vi "LV-Term UI.vi"(11 "LV-Term App In":refnum<class "LV-Term App.lvclass">) -> (3 "LV-Term App":refnum<class "LV-Term App.lvclass">)   [LabVIEW 2020, in "LV-Term App.lvclass"]
uses:
  LV-Term App.lvclass
  UI State.ctl
  LV-Term App.lvclass/LV-Term App.ctl
  Terminal/Terminal/Terminal.lvclass
  C:/Program Files (x86)/National Instruments/LabVIEW 2020/vi.lib/IlluminatedG/IG OOPanel/OOPanel/Panel/Panel.lvclass
  <vilib>/IlluminatedG/IG OOPanel/OOPanel/Manager/Manager.lvclass
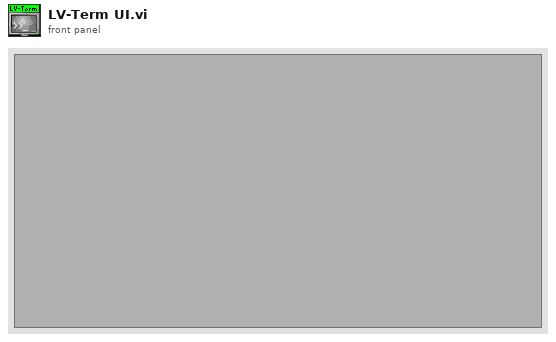
[diagram p1: front panel]
types:
  T1 = typedef "LV-Term App.lvclass/UI State.ctl" = enum16{"Init", "Run", "Close"}
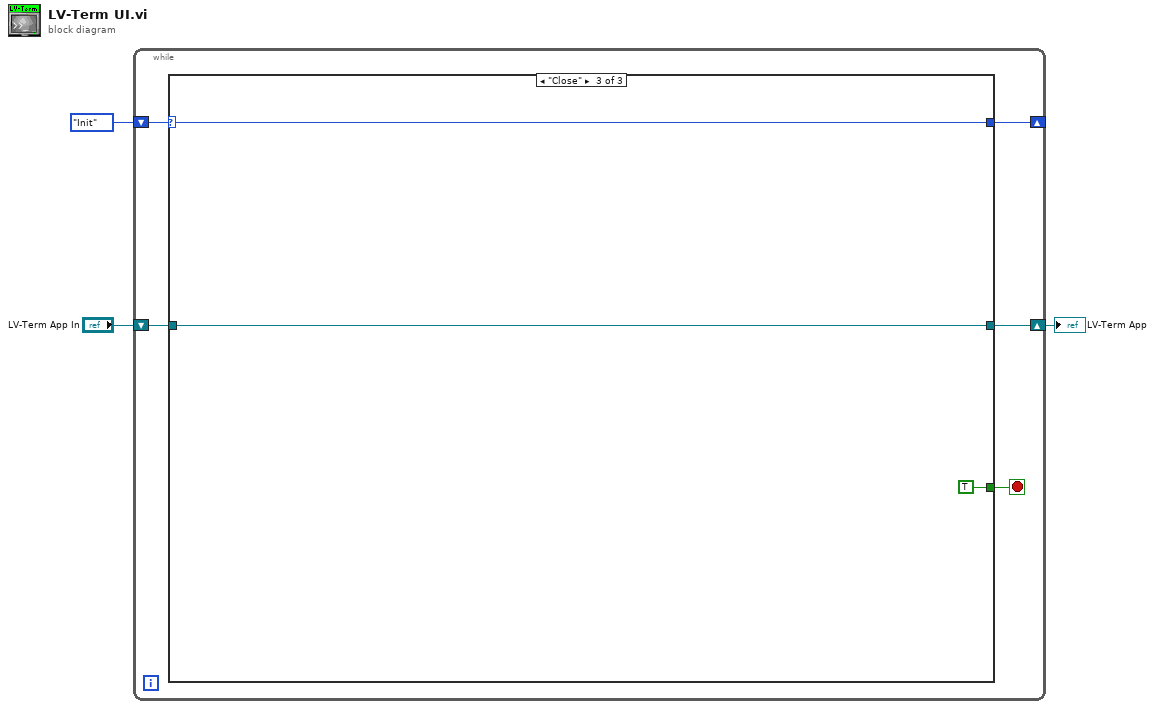
[diagram p0: block diagram]
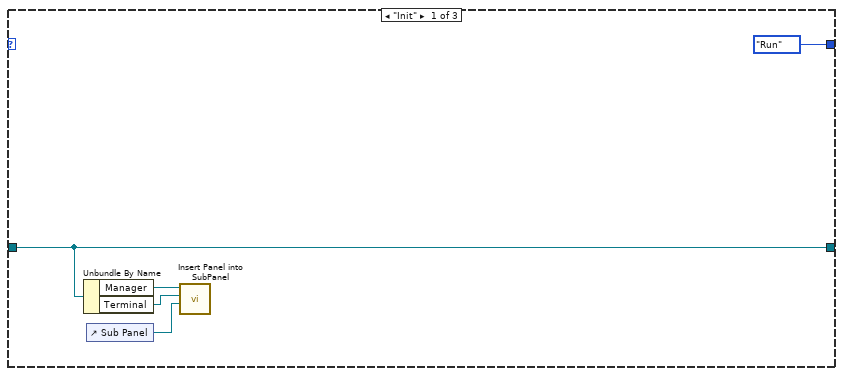
[diagram p2: hidden frame]
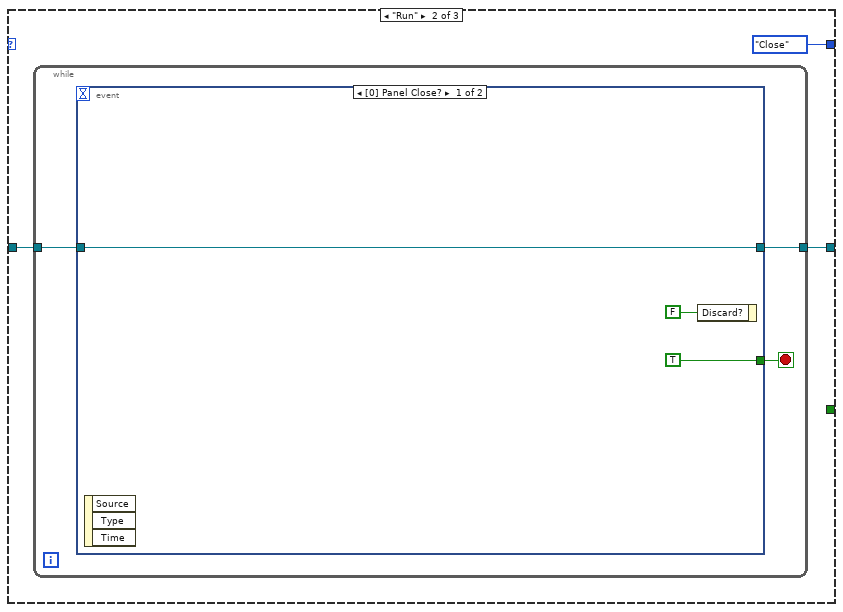
[diagram p3: hidden frame]
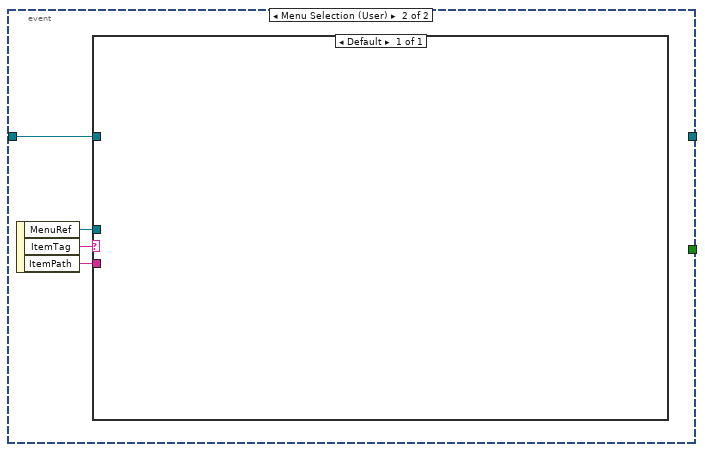
[diagram p4: hidden frame]
diagram:
  n1 = while {
    shift-right: [w7] -> _
    shift-left: UI_State."Init" ("UI State") -> [w8]
    shift-right: [w4] -> w1
    shift-left: "LV-Term App In" -> [w5]
    stop <- w6 stop-if-true
    n2 = case shown="\"Close\"" w8 {
      selector: w8 -> [_ _ w27]
      tunnel: [UI_State."Run" ("UI State") UI_State."Close" ("UI State") w27] -> w7
      tunnel: [_ _ TRUE] -> w6
      tunnel: w5 -> [w11 w15 w28]
      tunnel: [w11 w14 w28] -> w4
      frame "Init" {
        n3 = Unbundle By Name(w11) -> ("Manager"=w10:refnum<class "Manager.lvclass">, "Terminal"=w9:refnum<class "Terminal.lvclass">)
        n4 = control-ref of="Sub Panel"() -> (w12:refnum<vi>)
        n5 = call <vilib>:"Insert Panel into SubPanel.vi"("SubPanel"=w12, "Panel In"=w9, "Manager in"=w10) -> ()  [unwired: 6 in, 3 out]
      }
      frame "Run" {
        n6 = while {
          tunnel: w15 -> [w18]
          tunnel: [w17] -> w14
          stop <- w19 stop-if-true
          n7 = event shown="[0] Panel Close?" {
            selector: _ -> [_ _]
            dyn-events: _ -> [_ _]
            timeout: _ -> [_ _]
            tunnel: [TRUE ("Discard?") _] -> w19
            tunnel: w18 -> [w20 w23]
            tunnel: [w20 _] -> w17
            event Panel Close? {
              n8 = event-data() -> ()  [unwired: 1 in, 3 out]
              n9 = event-data("Discard?"=FALSE) -> ()  [unwired: 1 in, 1 out]
            }
            event Menu Selection (User) {
              n10 = event-data() -> ("MenuRef"=w25:refnum<k9>, "ItemTag"=w26:string, "ItemPath"=w24:string)  [unwired: 1 in]
              n11 = case shown="Default" w26 {
                tunnel: w25 -> [_]
                tunnel: w24 -> [_]
                tunnel: w23 -> [_]
                frame Default {
                }
              }
            }
          }
        }
      }
      frame "Close" {
      }
    }
  }
  "LV-Term App" <- w1
